vi "Create Master Instance (TCP).vi"(8 "error in (no error)":errorcluster caption="错误输入（无错误）", 10 "port (502)":u16=502 caption="端口(502)", 11 "address":string caption="地址") -> (0 "error out":errorcluster caption="错误输出", 3 "TCP master instance":refnum<class "Modbus Master.lvclass"> caption="TCP主设备实例")   [LabVIEW 2014, in "Modbus Master.lvclass"]
doc: "创建串口或TCPModbus主设备实例.必须手动选择所需多态实例。"
uses:
  <vilib>/Modbus/master/Modbus Master.lvclass
  <vilib>/Modbus/subvis/Transmission Data Unit (ADU)/IP Data Unit/IP Data Unit.lvclass
  <vilib>/Modbus/subvis/Protocol/TCP/TCP Master/TCP Master.lvclass
  <vilib>/Modbus/subvis/Protocol/TCP/TCP Master/TCP Master.lvclass/TCP Master.ctl
  <vilib>/Modbus/subvis/Transmission Data Unit (ADU)/Transmission Data Unit/Transmission Data Unit.lvclass/Transmission Data Unit.ctl
  <vilib>/Modbus/subvis/Modbus API/Modbus API.lvclass/Modbus API.ctl
  <vilib>/Modbus/master/Modbus Master.lvclass/Modbus Master.ctl
  <vilib>/Modbus/subvis/Protocol/TCP/TCP Master/Accessors/Address/Write Address.vi
  <vilib>/Modbus/subvis/Protocol/TCP/TCP Master/Accessors/Port/Write Port.vi
  <vilib>/Modbus/subvis/Modbus API/Modbus API.lvclass
  <vilib>/Modbus/subvis/Transmission Data Unit (ADU)/Transmission Data Unit/Transmission Data Unit.lvclass
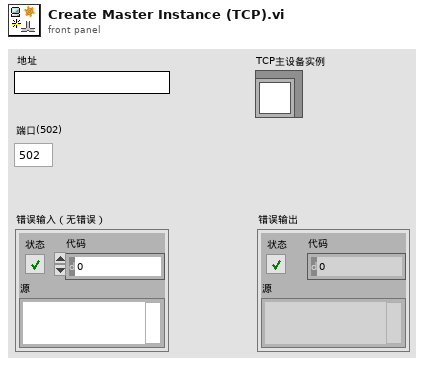
[diagram p1: front panel]
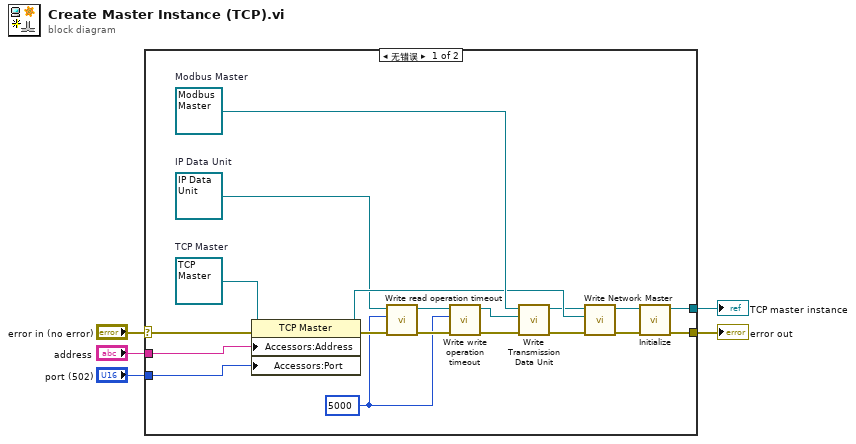
[diagram p0: block diagram]
diagram:
  n1 = case shown="无错误" "error in (no error)" {
    selector: "error in (no error)" -> [w8 w25]
    tunnel: "address" -> [w23 _]
    tunnel: "port (502)" -> [w22 _]
    tunnel: [w21 w25] -> w3
    tunnel: [w20 _] -> w2
    frame No Error {
      w9 = 5000 ("read operation timeout")
      w24 = refnum<class "TCP Master.lvclass"> refnum  # TCP Master
      w11 = refnum<class "IP Data Unit.lvclass"> refnum  # IP Data Unit
      w19 = refnum<class "Modbus Master.lvclass"> refnum  # Modbus Master
      n2 = property class="TCP Master"(reference=w24, error in=w8, "Accessors:Address"=w23, "Accessors:Port"=w22) -> (reference out=w18:refnum<class "TCP Master.lvclass">, error out=w10:errorcluster)
      n3 = call <vilib>:"Write read operation timeout.vi"("error in (no error)"=w10, "read operation timeout"=w9, "transmission data unit in"=w11) -> ("error out"=w14:errorcluster, "transmission data unit out"=w15:refnum<class "IP Data Unit.lvclass">)  [unwired: 7 in]
      n4 = call <vilib>:"Write write operation timeout.vi"("error in (no error)"=w14, "write operation timeout"=w9, "transmission data unit in"=w15) -> ("error out"=w13:errorcluster, "transmission data unit out"=w12:refnum<class "IP Data Unit.lvclass">)  [unwired: 7 in]
      n5 = call <vilib>:"Write Transmission Data Unit.vi"("error in (no error)"=w13, "transmission data unit"=w12, "Modbus instance in"=w19) -> ("error out"=w6:errorcluster, "Modbus instance out"=w7:refnum<class "Modbus Master.lvclass">)  [unwired: 7 in]
      n6 = call <vilib>:"Write Network Master.vi"("error in (no error)"=w6, "network master"=w18, "Modbus master in"=w7) -> ("error out"=w17:errorcluster, "Modbus master out"=w16:refnum<class "Modbus Master.lvclass">)  [unwired: 7 in]
      n7 = call-dynamic "Initialize.vi"("error in (no error)"=w17, "Modbus master in"=w16) -> ("error out"=w21:errorcluster, "Modbus master out"=w20:refnum<class "Modbus Master.lvclass">)  [unwired: 8 in]
    }
    frame Error {
    }
  }
  "error out" <- w3
  "TCP master instance" <- w2
